vi "Function_All.vi"(0 "Image Src":T3, 5 "Image Dst":T3, 7 "Pattern":T3, 9 "Data Array In":T2, 11 "Error in":errorcluster) -> (4 "Result Array Out":T1(array[cluster]), 15 "Error Out":errorcluster)   [LabVIEW 2013]
uses:
  <vilib>/vision/Image Controls.llb/IMAQ Image.ctl
  Control/Control_Data Array.ctl
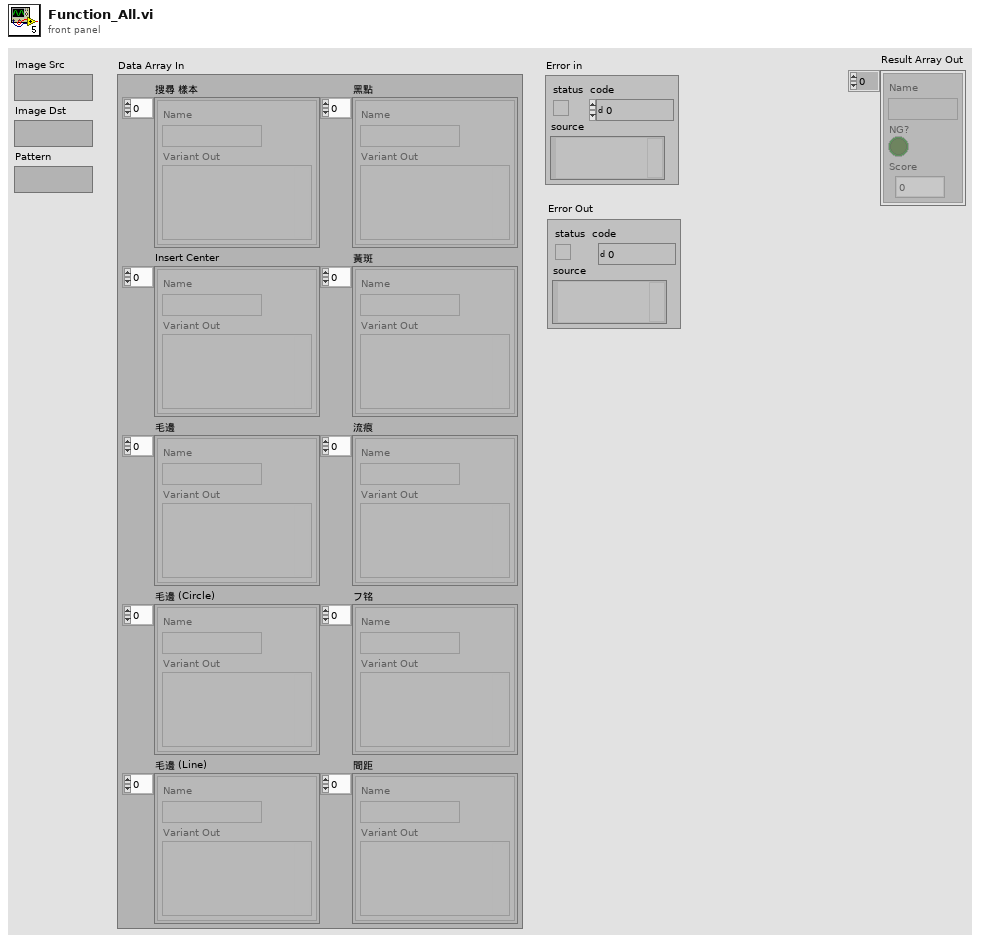
[diagram p1: front panel]
types:
  T1 = cluster{"Name":string, "NG?":bool, "Score":dbl}[]
  T2 = typedef "Control_Data Array.ctl" = cluster{"搜尋 樣本":cluster{"Name":string, "Variant Out":variant}[], "Insert Center":cluster{"Name":string, "Variant Out":variant}[], "毛邊":cluster{"Name":string, "Variant Out":variant}[], "毛邊 (Circle)":cluster{"Name":string, "Variant Out":variant}[], "毛邊 (Line)":cluster{"Name":string, "Variant Out":variant}[], "黑點":cluster{"Name":string, "Variant Out":variant}[], "黃斑":cluster{"Name":string, "Variant Out":variant}[], "流痕":cluster{"Name":string, "Variant Out":variant}[], "フ铭":cluster{"Name":string, "Variant Out":variant}[], "間距":cluster{"Name":string, "Variant Out":variant}[]}
  T3 = typedef "IMAQ Image.ctl" = refnum<image>
  T4 = typedef "IMAQ Coordinate System" = cluster{"Reference System":cluster{"Origin":cluster{"X":sgl, "Y":sgl}, "Angle (deg)":sgl, "Axis Reference":u32}, "Measurement System":cluster{"Origin":cluster{"X":sgl, "Y":sgl}, "Angle (deg)":sgl, "Axis Reference":u32}}
  T5 = cluster{"Position":cluster{"x":sgl, "y":sgl}, "Angle":sgl, "Scale":sgl, "Score":sgl, "Bounding Box":cluster{"x":sgl, "y":sgl}[]}[]
  T6 = cluster{"Max Position":cluster{"X":sgl, "Y":sgl}, "Min Position":cluster{"X":sgl, "Y":sgl}}
  T7 = cluster{"Center":cluster{"X":sgl, "Y":sgl}, "Diameter":dbl, "Max value":sgl, "min value":sgl}
  T8 = cluster{"Start Point":cluster{"X":i32, "Y":i32}, "End Point":cluster{"X":i32, "Y":i32}}
  T9 = cluster{"Show Search Area":bool, "Show Center":bool, "Show Bounding Box":bool}
  T10 = cluster{"Object Center":cluster{"X":dbl, "Y":dbl}, "Bounding Box":cluster{"X Left":dbl, "Y Top":dbl, "X Right":dbl, "Y Bottom":dbl}, "Area":dbl}[]
  T11 = cluster{"Global Rectangle":i32[], "Contours":cluster{"ID":enum32{"External", "Internal"}, "Type":u32, "Coordinates":i32[]}[]}
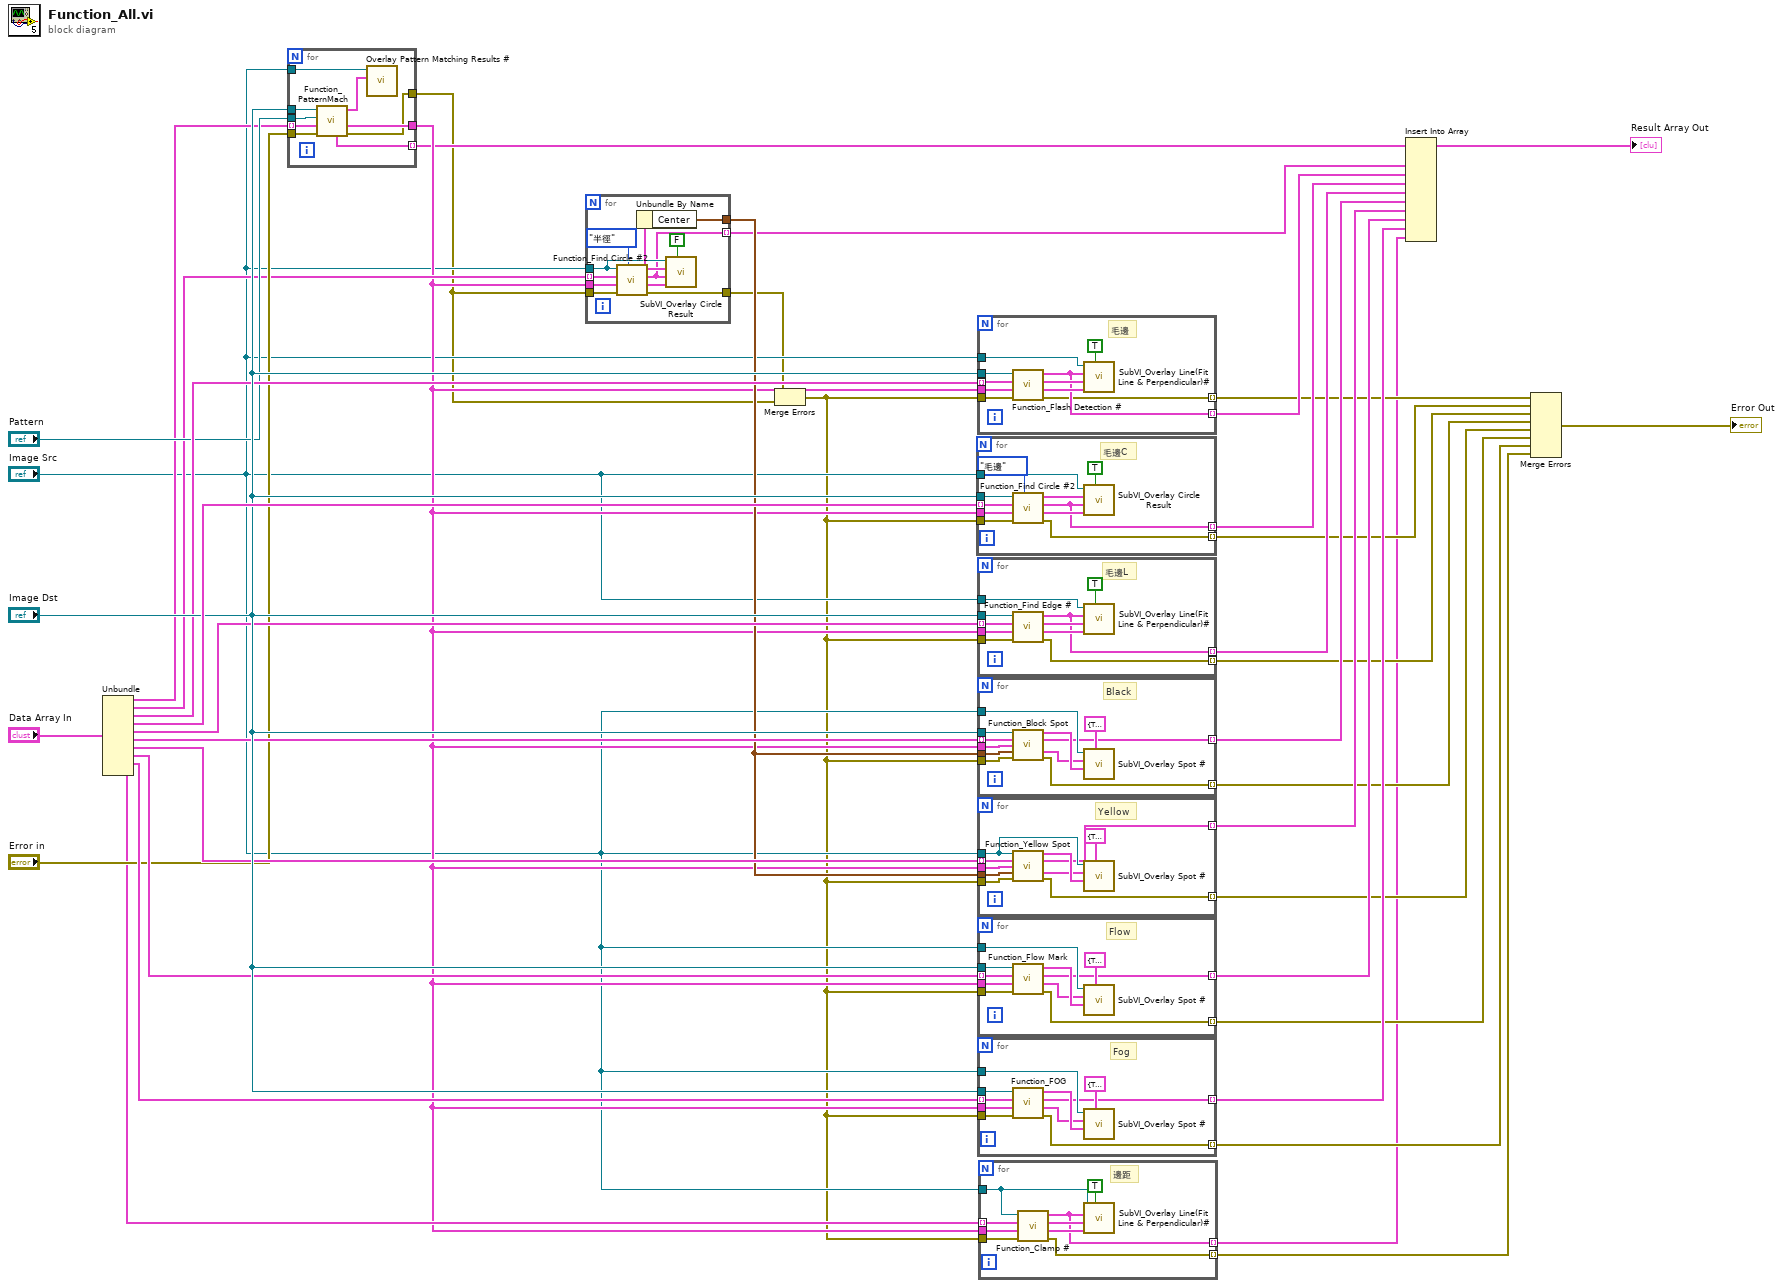
[diagram p0: block diagram]
diagram:
  n1 = Unbundle("Data Array In") -> ("搜尋 樣本"=w12:cluster{"Name":string, "Variant Out":variant}[], "Insert Center"=w13:cluster{"Name":string, "Variant Out":variant}[], "毛邊"=w37:cluster{"Name":string, "Variant Out":variant}[], "毛邊 (Circle)"=w40:cluster{"Name":string, "Variant Out":variant}[], "毛邊 (Line)"=w38:cluster{"Name":string, "Variant Out":variant}[], "黑點"=w33:cluster{"Name":string, "Variant Out":variant}[], "黃斑"=w32:cluster{"Name":string, "Variant Out":variant}[], "流痕"=w35:cluster{"Name":string, "Variant Out":variant}[], "フ铭"=w36:cluster{"Name":string, "Variant Out":variant}[], "間距"=w9:cluster{"Name":string, "Variant Out":variant}[])
  n2 = for {
    tunnel: [w49] -> w8
    tunnel: "Image Dst" -> [w48]
    tunnel: "Pattern" -> [w47]
    tunnel: w12 -> [w46] mode=indexing
    tunnel: "Error in" -> [w44]
    tunnel: [w43] -> w4 mode=indexing
    tunnel: "Image Src" -> [w42]
    tunnel: [w41] -> w1
    n3 = call "Function_PatternMach.vi"("Error in"=w44, "Data Cluster In"=w46, "Template Image"=w47, "Image Src In"=w48) -> ("Error out"=w41:errorcluster, "CoordSys Out"=w49:T4, "Matches"=w45:T5, "Result(PM)"=w43:cluster{"Name":string, "NG?":bool, "Score":dbl})  [unwired: 3 in, 1 out]
    n4 = call "Overlay Pattern Matching Results #.vi"("Matches"=w45, "Image"=w42) -> ()  [unwired: 8 in, 2 out]
  }
  n5 = for {
    tunnel: w8 -> [w60]
    tunnel: [w59] -> w31
    tunnel: w13 -> [w58] mode=indexing
    tunnel: "Image Src" -> [w54]
    tunnel: w1 -> [w53]
    tunnel: [w52] -> w3
    tunnel: [w51] -> w14 mode=indexing
    n6 = call "Function_Find Circle #2.vi"("功能"=enum16{"半徑", "毛邊"}."半徑", "Error in"=w53, "CoordSys In"=w60, "Data Cluster In"=w58, "Image Src"=w54) -> ("Error Out"=w52:errorcluster, "Max & min"=w55:T6, "Result(Circ)"=w51:cluster{"Name":string, "NG?":bool, "Score":dbl}, "Result"=w56:T7)  [unwired: 2 in, 1 out]
    n7 = Unbundle By Name(w56) -> ("Center"=w59:cluster{"X":sgl, "Y":sgl})
    n8 = call "SubVI_Overlay Circle Result.vi"("Overlay Result"=FALSE, "Max & min"=w55, "Result"=w51, "Result In"=w56, "Image"=w54) -> ()  [unwired: 7 in]
  }
  n9 = Merge Errors(w3, w1) -> (w2:errorcluster)
  n10 = for {
    tunnel: "Image Dst" -> [w69]
    tunnel: "Image Src" -> [w68]
    tunnel: w40 -> [w67] mode=indexing
    tunnel: w8 -> [w66]
    tunnel: [w62] -> w28 mode=indexing
    tunnel: w2 -> [w64]
    tunnel: [w63] -> w20 mode=indexing
    # "毛邊C"
    n11 = call "Function_Find Circle #2.vi"("功能"=enum16{"半徑", "毛邊"}."毛邊", "Error in"=w64, "CoordSys In"=w66, "Data Cluster In"=w67, "Image Src"=w69) -> ("Error Out"=w63:errorcluster, "Max & min"=w70:T6, "Result(Circ)"=w62:cluster{"Name":string, "NG?":bool, "Score":dbl}, "Result"=w65:T7)  [unwired: 2 in, 1 out]
    n12 = call "SubVI_Overlay Circle Result.vi"("Overlay Result"=TRUE, "Max & min"=w70, "Result"=w62, "Result In"=w65, "Image"=w68) -> ()  [unwired: 7 in]
  }
  n13 = for {
    tunnel: "Image Dst" -> [w81]
    tunnel: w37 -> [w80] mode=indexing
    tunnel: w8 -> [w79]
    tunnel: "Image Src" -> [w77]
    tunnel: [w74] -> w22 mode=indexing
    tunnel: w2 -> [w73]
    tunnel: [w72] -> w21 mode=indexing
    # "毛邊"
    n14 = call "Function_Flash Detection #.vi"("Error in"=w73, "CoordSys In"=w79, "Data Cluster In"=w80, "Image Dst In"=w81) -> ("Error out"=w72:errorcluster, "Perpendicular Line(Offset)"=w75:T8, "Fit Line(Offset)"=w76:T8, "Result(Flash)"=w74:cluster{"Name":string, "NG?":bool, "Score":dbl})  [unwired: 3 in, 1 out]
    n15 = call "SubVI_Overlay Line(Fit Line & Perpendicular)#.vi"("Overlay Result"=TRUE, "Perpendicular Line(Offset)"=w75, "Fit Line(Offset)"=w76, "Result"=w74, "Image Src In"=w77) -> ()  [unwired: 7 in]
  }
  n16 = for {
    tunnel: "Image Dst" -> [w85]
    tunnel: w38 -> [w86] mode=indexing
    tunnel: w8 -> [w87]
    tunnel: "Image Src" -> [w90]
    tunnel: [w84] -> w27 mode=indexing
    tunnel: w2 -> [w83]
    tunnel: [w82] -> w19 mode=indexing
    # "毛邊L"
    n17 = call "Function_Find Edge #.vi"("Error in"=w83, "CoordSys In"=w87, "Data Cluster In"=w86, "Image Src"=w85) -> ("Error Out"=w82:errorcluster, "Perpendicular Line(Offset)"=w88:T8, "Fit Line(Offset)"=w89:T8, "Result"=w84:cluster{"Name":string, "NG?":bool, "Score":dbl})  [unwired: 3 in, 1 out]
    n18 = call "SubVI_Overlay Line(Fit Line & Perpendicular)#.vi"("Overlay Result"=TRUE, "Perpendicular Line(Offset)"=w88, "Fit Line(Offset)"=w89, "Result"=w84, "Image Src In"=w90) -> ()  [unwired: 7 in]
  }
  n19 = for {
    tunnel: w31 -> [w102]
    tunnel: w33 -> [w101] mode=indexing
    tunnel: w8 -> [w100]
    tunnel: "Image Src" -> [w96]
    tunnel: [w95] -> w26 mode=indexing
    tunnel: "Image Dst" -> [w94]
    tunnel: w2 -> [w93]
    tunnel: [w92] -> w18 mode=indexing
    # "Black"
    n20 = call "Function_Block Spot.vi"("Image Dst In"=w94, "Data Cluster In"=w101, "CoordSys In"=w100, "Center(Annulus)"=w102, "Error in"=w93) -> ("Objects"=w98:T10, "Result(Black)"=w95:cluster{"Name":string, "NG?":bool, "Score":dbl}, "ROI Out"=w97:T11, "Error out"=w92:errorcluster)  [unwired: 6 in, 1 out]
    n21 = call "SubVI_Overlay Spot #.vi"("Setup"=T9 {"Show Search Area"=TRUE, "Show Center"=TRUE, "Show Bounding Box"=TRUE}, "Objects"=w98, "ROI"=w97, "Image In"=w96) -> ()  [unwired: 6 in, 2 out]
  }
  n22 = for {
    tunnel: w31 -> [w112]
    tunnel: w32 -> [w111] mode=indexing
    tunnel: w8 -> [w110]
    tunnel: "Image Src" -> [w106]
    tunnel: [w105] -> w25 mode=indexing
    tunnel: w2 -> [w104]
    tunnel: [w103] -> w17 mode=indexing
    # "Yellow"
    n23 = call "Function_Yellow Spot.vi"("Image Src In"=w106, "Data Cluster In"=w111, "CoordSys In"=w110, "Center(Annulus)"=w112, "Error in"=w104) -> ("Objects"=w108:T10, "Result(Yellow)"=w105:cluster{"Name":string, "NG?":bool, "Score":dbl}, "ROI Out"=w107:T11, "Error out"=w103:errorcluster)  [unwired: 6 in, 1 out]
    n24 = call "SubVI_Overlay Spot #.vi"("Setup"=T9 {"Show Search Area"=TRUE, "Show Center"=TRUE, "Show Bounding Box"=TRUE}, "Objects"=w108, "ROI"=w107, "Image In"=w106) -> ()  [unwired: 6 in, 2 out]
  }
  n25 = for {
    tunnel: w35 -> [w116] mode=indexing
    tunnel: "Image Src" -> [w121]
    tunnel: [w118] -> w24 mode=indexing
    tunnel: "Image Dst" -> [w120]
    tunnel: w8 -> [w115]
    tunnel: w2 -> [w114]
    tunnel: [w113] -> w16 mode=indexing
    # "Flow"
    n26 = call "Function_Flow Mark.vi"("Error in"=w114, "CoordSys In"=w115, "Data Cluster In"=w116, "Image Dst In"=w120) -> ("Error out"=w113:errorcluster, "ROI Out"=w117:T11, "Result(Flow Mark)"=w118:cluster{"Name":string, "NG?":bool, "Score":dbl}, "Objects"=w119:T10)  [unwired: 3 in, 1 out]
    n27 = call "SubVI_Overlay Spot #.vi"("Setup"=T9 {"Show Search Area"=TRUE, "Show Center"=TRUE, "Show Bounding Box"=TRUE}, "Objects"=w119, "ROI"=w117, "Image In"=w121) -> ()  [unwired: 6 in, 2 out]
  }
  n28 = for {
    tunnel: w36 -> [w126] mode=indexing
    tunnel: "Image Src" -> [w131]
    tunnel: [w128] -> w23 mode=indexing
    tunnel: "Image Dst" -> [w130]
    tunnel: w8 -> [w125]
    tunnel: w2 -> [w124]
    tunnel: [w123] -> w15 mode=indexing
    # "Fog"
    n29 = call "Function_FOG.vi"("Error in"=w124, "CoordSys In"=w125, "Data Cluster In"=w126, "Image Dst In"=w130) -> ("Error out"=w123:errorcluster, "ROI Out"=w127:T11, "Result(Black)"=w128:cluster{"Name":string, "NG?":bool, "Score":dbl}, "Objects"=w129:T10)  [unwired: 3 in, 1 out]
    n30 = call "SubVI_Overlay Spot #.vi"("Setup"=T9 {"Show Search Area"=TRUE, "Show Center"=TRUE, "Show Bounding Box"=TRUE}, "Objects"=w129, "ROI"=w127, "Image In"=w131) -> ()  [unwired: 6 in, 2 out]
  }
  n31 = for {
    tunnel: w9 -> [w139] mode=indexing
    tunnel: [w136] -> w6 mode=indexing
    tunnel: w8 -> [w138]
    tunnel: "Image Src" -> [w135]
    tunnel: [w134] -> w5 mode=indexing
    tunnel: w2 -> [w133]
    # "邊距"
    n32 = call "Function_Clamp #.vi"("Error in"=w133, "CoordSys In"=w138, "Data Cluster In"=w139, "Image Src"=w135) -> ("Error Out"=w136:errorcluster, "Perpendicular Line(Offset)"=w141:T8, "Fit Line(Offset)"=w137:T8, "Result"=w134:cluster{"Name":string, "NG?":bool, "Score":dbl})  [unwired: 3 in, 1 out]
    n33 = call "SubVI_Overlay Line(Fit Line & Perpendicular)#.vi"("Overlay Result"=TRUE, "Perpendicular Line(Offset)"=w141, "Fit Line(Offset)"=w137, "Result"=w134, "Image Src In"=w135) -> ()  [unwired: 7 in]
  }
  n34 = Insert Into Array(array=w4, new element #1=w14, new element #2=w22, new element #3=w28, new element #4=w27, new element #5=w26, new element #6=w25, new element #7=w24, new element #8=w23, new element #9=w5) -> (→"Result Array Out":T1)  [unwired: 1 in]
  n35 = Merge Errors(w21, w20, w19, w18, w17, w16, w15, w6) -> (→"Error Out":errorcluster)
